vi "ELYSE_clock_pulses.vi"(6 "pulses previous":dbl, 8 "error in (no error)":errorcluster caption="entrée d'erreur (pas d'erreur)", 9 "ControlQueue":refnum<queue>, 10 "divider":dbl, 11 "DAQmxTaskContainer en entrée":refnum<class "DAQmxTaskContainer.lvclass">) -> (0 "error out":errorcluster caption="sortie d'erreur", 2 "pulses":dbl, 3 "DAQmxTaskContainer en sortie":refnum<class "DAQmxTaskContainer.lvclass">)   [LabVIEW 2015, in "DAQmxTaskContainer.lvclass"]
uses:
  DAQmxTaskContainer.lvclass
  DAQmxTaskContainer_General/DAQmxTaksContainer_General.lvclass/DAQmxTaksContainer_General.ctl
  dependecies/ControlsVIs/Clusters-def/Standard Command.ctl
  dependecies/ControlsVIs/Clusters-def/DAQmx-ELYSE_pulse_counter.ctl
  dependecies/ControlsVIs/Clusters-def/SERVER-Commands.ctl
  DAQmxTask.lvclass
  DAQmxTaskContainer_General/DAQmxTaksContainer_General.lvclass
  Control/Control-Server/Control-Server.lvclass
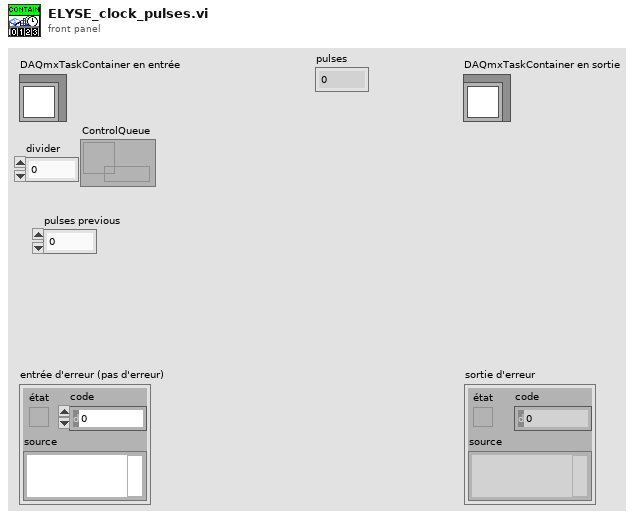
[diagram p1: front panel]
types:
  T1 = typedef "DAQmxTaksContainer_General.lvclass/DAQmx-ELYSE_pulse_counter.ctl" = cluster{"# counts":dbl}
  T2 = typedef "Standard Command.ctl" = cluster{"command":string, "data":variant}
  T3 = typedef "Control-Server.lvclass/SERVER-Commands.ctl" = string
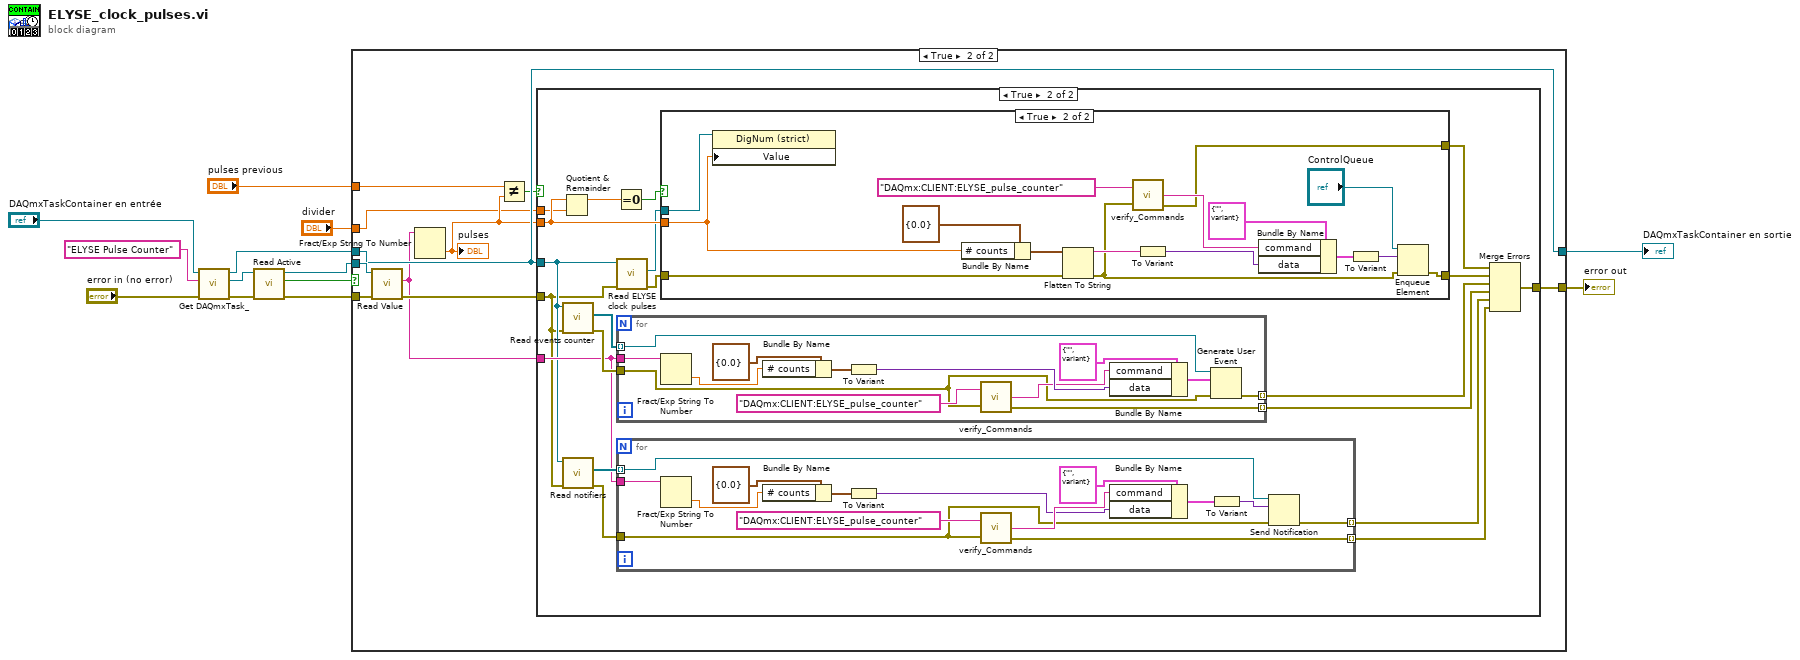
[diagram p0: block diagram]
diagram:
  n1 = call "Get DAQmxTask_.vi"("error in (no error)"="error in (no error)", "Task name"="ELYSE Pulse Counter", "DAQmxTaksContainer_General in"="DAQmxTaskContainer en entrée") -> ("error out"=w10:errorcluster, "DAQmx Task"=w7:refnum<class "DAQmxTask.lvclass">, "DAQmxTaksContainer_General out"=w3:refnum<class "DAQmxTaskContainer.lvclass">)  [unwired: 6 in]
  n2 = call-dynamic "Read Active.vi"("error in (no error)"=w10, "DAQmxTask in"=w7) -> ("error out"=w9:errorcluster, "Active?"=w8:bool, "DAQmxTask out"=w6:refnum<class "DAQmxTask.lvclass">)  [unwired: 7 in]
  n3 = case shown="True" w8 {
    tunnel: w3 -> [w14 w21]
    tunnel: w9 -> [w15 w25]
    tunnel: w6 -> [_ w24]
    tunnel: [w14 w21] -> w5
    tunnel: [w15 w23] -> w4
    tunnel: "pulses previous" -> [_ w18]
    tunnel: "divider" -> [_ w16]
    frame False {
    }
    frame True {
      n4 = call-dynamic "Read Value.vi"("error in (no error)"=w25, "DAQmxTask en entrée"=w24) -> ("error out"=w22:errorcluster, "Data string"=w20:string)  [unwired: 6 in, 2 out]
      n5 = Fract/Exp String To Number(string=w20) -> (number=w17:dbl)  [unwired: 3 in, 1 out]
      "pulses" <- w17
      n6 = Not Equal?(x=w18, y=w17) -> (x != y?=w19:bool)
      n7 = case shown="True" w19 {
        tunnel: [w26 w42] -> w23
        tunnel: w22 -> [w26 w29]
        tunnel: w21 -> [_ w30]
        tunnel: w20 -> [_ w35]
        tunnel: w17 -> [_ w32]
        tunnel: w16 -> [_ w27]
        frame False {
        }
        frame True {
          n8 = Quotient & Remainder(x=w32, y=w27) -> (x-y*floor(x/y)=w46:dbl)  [unwired: 1 out]
          n9 = call "Read events counter.vi"("error in (no error)"=w29, "DAQmxTaksContainer_General in"=w30) -> ("error out"=w41:errorcluster, "events counter"=w44:refnum<user-event>[])  [unwired: 7 in, 1 out]
          n10 = call "Read notifiers.vi"("error in (no error)"=w29, "DAQmxTaksContainer_General in"=w30) -> ("error out"=w37:errorcluster, "notifiers"=w36:refnum<notifier>[])  [unwired: 7 in, 1 out]
          n11 = Equal To 0?(x=w46) -> (x = 0?=w45:bool)
          n12 = call "Read ELYSE clock pulses.vi"("error in (no error)"=w29, "DAQmxTaksContainer_General in"=w30) -> ("error out"=w28:errorcluster, "ELYSE clock pulses"=w31:refnum<vi>)  [unwired: 7 in, 1 out]
          n13 = for {
            tunnel: w35 -> [w72]
            tunnel: w41 -> [w62]
            tunnel: w44 -> [w69] mode=indexing
            tunnel: [w68] -> w43 mode=indexing
            tunnel: [w61] -> w38 mode=indexing
            n14 = Fract/Exp String To Number(string=w72) -> (number=w67:dbl)  [unwired: 3 in, 1 out]
            n15 = Bundle By Name(cluster=T1 {"# counts"=0.0} ("OSc:Read"), "# counts"=w67) -> (w66:T1)
            n16 = To Variant(anything=w66) -> (Variant=w65:variant)
            n17 = call "verify_Commands.vi"("Command"="DAQmx:CLIENT:ELYSE_pulse_counter" ("command"), "error in"=w62) -> ("Command out"=w63:string, "error out"=w61:errorcluster)  [unwired: 1 out]
            n18 = Bundle By Name(cluster=T2 {"command"="", "data"=variant} ("command"), "command"=w63, "data"=w65) -> (w71:T2)
            n19 = Generate User Event(user event=w69, event data cluster=w71, error in=w62) -> (error out=w68:errorcluster)  [unwired: 1 in, 1 out]
          }
          n20 = for {
            tunnel: w37 -> [w48]
            tunnel: w36 -> [w51] mode=indexing
            tunnel: w35 -> [w53]
            tunnel: [w52] -> w33 mode=indexing
            tunnel: [w47] -> w34 mode=indexing
            n21 = Fract/Exp String To Number(string=w53) -> (number=w56:dbl)  [unwired: 3 in, 1 out]
            n22 = Bundle By Name(cluster=T1 {"# counts"=0.0} ("OSc:Read"), "# counts"=w56) -> (w57:T1)
            n23 = To Variant(anything=w57) -> (Variant=w58:variant)
            n24 = call "verify_Commands.vi"("Command"="DAQmx:CLIENT:ELYSE_pulse_counter" ("command"), "error in"=w48) -> ("Command out"=w60:string, "error out"=w52:errorcluster)  [unwired: 1 out]
            n25 = Bundle By Name(cluster=T2 {"command"="", "data"=variant} ("command"), "command"=w60, "data"=w58) -> (w50:T2)
            n26 = To Variant(anything=w50) -> (Variant=w49:variant)
            n27 = Send Notification(notification=w49, notifier=w51, error in (no error)=w48) -> (error out=w47:errorcluster)  [unwired: 1 out]
          }
          n28 = case shown="True" w45 {
            tunnel: w31 -> [_ w90]
            tunnel: w32 -> [_ w88]
            tunnel: w28 -> [w74 w81]
            tunnel: [w74 w80] -> w40
            tunnel: [_ w75] -> w39
            frame False {
            }
            frame True {
              n29 = property class="DigNum (strict)"(reference=w90, "Value"=w88) -> ()  [unwired: 1 in, 2 out]
              n30 = Bundle By Name(cluster=T1 {"# counts"=0.0} ("OSc:Read"), "# counts"=w88) -> (w82:T1)
              n31 = Flatten To String(anything=w82, error in (no error)=w81) -> (data string=w85:string, error out=w76:errorcluster)  [unwired: 2 in, 1 out]
              n32 = call "verify_Commands.vi"("Command"=T3 "DAQmx:CLIENT:ELYSE_pulse_counter" ("Commands"), "error in"=w76) -> ("Command out"=w77:string, "error out"=w75:errorcluster)  [unwired: 1 out]
              n33 = To Variant(anything=w85) -> (Variant=w84:variant)
              n34 = Bundle By Name(cluster=T2 {"command"="", "data"=variant} ("input cluster"), "command"=w77, "data"=w84) -> (w83:T2)
              n35 = To Variant(anything=w83) -> (Variant=w87:variant)
              n36 = Enqueue Element(queue="ControlQueue", element=w87, error in (no error)=w76) -> (error out=w80:errorcluster)  [unwired: 1 in, 2 out]
            }
          }
          n37 = Merge Errors(w39, w40, w43, w38, w34, w33) -> (w42:errorcluster)
        }
      }
    }
  }
  "DAQmxTaskContainer en sortie" <- w5
  "error out" <- w4
